vi "RemoveConnectID for PicoPadServer.vi"(8 "ConnectArrayIN":T1(array[cluster]), 11 "ConnectID":refnum<k5>) -> (0 "ConnectArrayOUT":T1(array[cluster]))   [LabVIEW 2011]
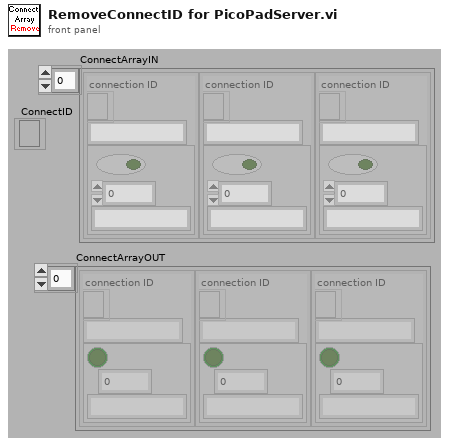
[diagram p1: front panel]
types:
  T1 = cluster{"connection ID":refnum<k5>, string, errorcluster}[]
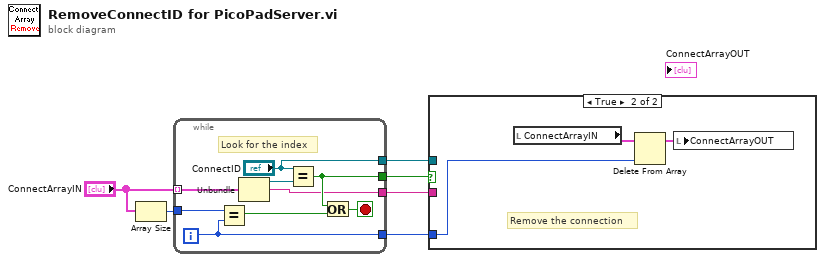
[diagram p0: block diagram]
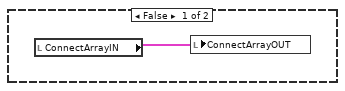
[diagram p2: hidden frame]
diagram:
  n1 = Array Size(array="ConnectArrayIN") -> (size(s)=w5:i32)
  n2 = while {
    tunnel: "ConnectArrayIN" -> [w15] mode=indexing
    tunnel: w5 -> [w12]
    tunnel: [w10] -> w4
    tunnel: [w9] -> w3
    tunnel: [w8] -> w2
    tunnel: ["ConnectID"] -> w1
    i -> [w9]
    stop <- w11 stop-if-true
    # "Look for the index"
    n3 = Equal?(x=w12, y=w9) -> (x = y?=w13:bool)
    n4 = Unbundle(w15) -> ("connection ID"=w14:refnum<k5>, w8:string)  [unwired: 1 out]
    n5 = Equal?(x="ConnectID", y=w14) -> (x = y?=w10:bool)
    n6 = Or(x=w10, y=w13) -> (x .or. y?=w11:bool)
  }
  n7 = case shown="True" w4 {
    tunnel: w3 -> [_ w17]
    tunnel: w2 -> [_ _]
    tunnel: w1 -> [_ _]
    frame False {
      n8 = local read "ConnectArrayIN"() -> (w16:T1)
      n9 = local write "ConnectArrayOUT"(w16) -> ()
    }
    frame True {
      # "Remove the connection"
      n10 = local read "ConnectArrayIN"() -> (w19:T1)
      n11 = Delete From Array(array=w19, index=w17) -> (array with subset deleted=w18:T1)  [unwired: 1 in, 1 out]
      n12 = local write "ConnectArrayOUT"(w18) -> ()
    }
  }
